vi "Initialize.vi"(8 "error in":errorcluster, 9 "PPLs Folder Path":path, 10 "INI File Path":path, 11 "Device":string) -> (0 "error out":errorcluster, 3 "Axis out":refnum<class "Axis.lvclass">)   [LabVIEW 2018, in "Axis.lvlib" / "Axis.lvclass"]
uses:
  Axis.lvclass
  Custom Controls/Command.ctl
  Axis.lvclass/Axis.ctl
  PPLs/Configuration/Configuration.lvlibp/Configuration.lvclass
  Axis.lvlib
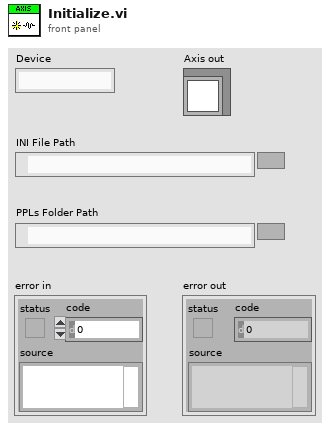
[diagram p1: front panel]
types:
  T1 = typedef "Axis.lvlib/Command.ctl" = enum16{"None", "Home", "Renumber", "Move Absolute", "Move Relative", "Stop", "Set Run Speed", "Set Acceleration", "Set Run Current", "Set Home Offset", "Set Home Speed", "Query Current Position", "Load Defaults", "Query Status", "Lock Controls", "Unlock Controls", "Set Jog Step Size", "Set Jog Acceleration", "Set Jog Speed", "Query Homed Status", "Query Moving Status", "Reset", "Set Max Position", "Set Min Position"}
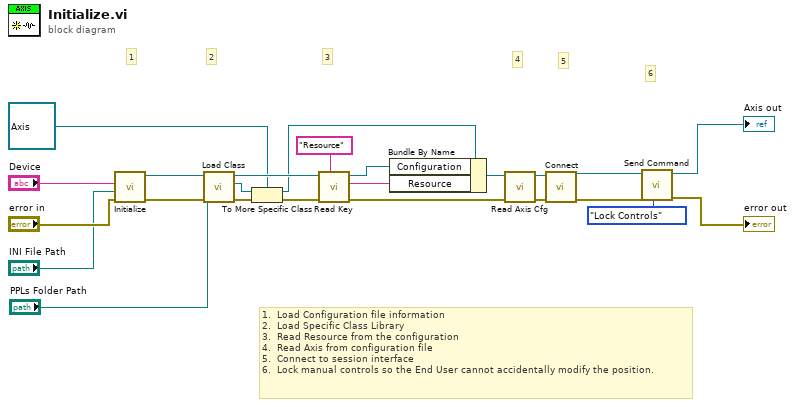
[diagram p0: block diagram]
diagram:
  # "1.  Load Configuration file information\n2.  Load Specific Class Library\n3.  Read Resource from the configuration\n4.  Read Axis from configuration file\n5.  Connect to session interface\n6.  Lock manual controls so the End User cannot accidentally modify the position."
  # "6"
  # "5"
  # "4"
  # "3"
  # "2"
  # "1"
  n1 = call "Initialize.vi"("error in"="error in", "INI File Path"="INI File Path", "Device"="Device") -> ("error out"=w22:errorcluster, "Configuration out"=w23:refnum<class "Configuration.lvclass">)  [unwired: 7 in]
  n2 = call "Load Class.vi"("error in"=w22, "PPLs Folder Path"="PPLs Folder Path", "Configuration in"=w23) -> ("error out"=w21:errorcluster, "Class out"=w20:refnum<class>, "Configuration out"=w19:refnum<class "Configuration.lvclass">)  [unwired: 6 in]
  n3 = To More Specific Class(target class=refnum<class "Axis.lvclass"> refnum ("Axis in"), reference=w20, error in=w21) -> (specific class reference=w16:refnum<class "Axis.lvclass">, error out=w18:errorcluster)
  n4 = call "Read Key.vi"("Key:"="Resource", "error in"=w18, "Configuration in"=w19) -> ("error out"=w8:errorcluster, "Value"=w15:string, "Configuration out"=w12:refnum<class "Configuration.lvclass">)  [unwired: 6 in]
  n5 = Bundle By Name(cluster=w16, "Configuration"=w12, "Resource"=w15) -> (w11:refnum<class "Axis.lvclass">)
  n6 = call "Read Axis Cfg.vi"("error in (no error)"=w8, "Axis in"=w11) -> ("error out"=w9:errorcluster, "Axis out"=w10:refnum<class "Axis.lvclass">)  [unwired: 8 in]
  n7 = call-dynamic "Connect.vi"("error in"=w9, "Axis in"=w10) -> ("error out"=w4:errorcluster, "Axis out"=w3:refnum<class "Axis.lvclass">)  [unwired: 8 in]
  n8 = call-dynamic "Send Command.vi"("Command"=Command."Lock Controls", "error in"=w4, "Axis in"=w3) -> ("error out"=→"error out":errorcluster, "Axis out"=→"Axis out":refnum<class "Axis.lvclass">)  [unwired: 7 in]
